vi "Signal.vi"() -> ()   [LabVIEW 2017]
uses:
  <vilib>/measure/NI_MABase.lvlib
panel:
  out "Waveform Chart":dynamicdata(graph)
  in  "sampling info":cluster{"Fs":dbl, "#s":dbl}={"Fs"=1000.0, "#s"=1000.0} {"Fs" format="%.2p"}
  out "data 2":waveform(dbl)(graph) caption="data"
  in  "Desviación\nEstandar":dbl=1.0 format="%.2p"
  in  "input cluster":T1={"amplitude"=2.0, "frequency"=10.0, "offset"=2.0, "square wave duty cycle (%)"=50.0, "reset signal"=FALSE, "signal type"=enum."Sine Wave", "phase"=0.0} {"phase" format="%.2p"; "square wave duty cycle (%)" format="%0.2f"; "offset" format="%0.2p"; "frequency" format="%0.2p"; "amplitude" format="%0.2p"}
  in  "device name":tag="myDAQ1"
  out "data":dynamicdata(graph)
  in  "stop":bool
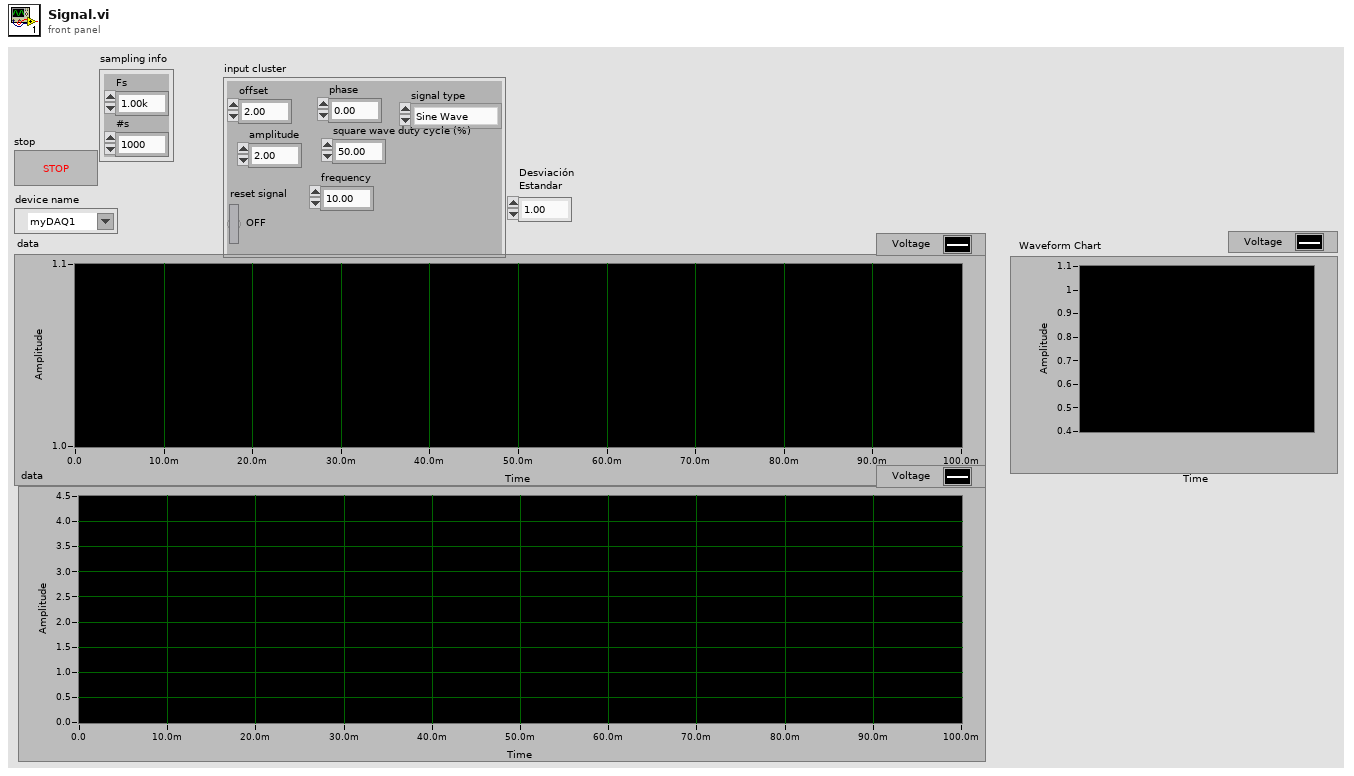
[diagram p1: front panel]
types:
  T1 = cluster{"amplitude":dbl, "frequency":dbl, "offset":dbl, "square wave duty cycle (%)":dbl, "reset signal":bool, "signal type":enum16{"Sine Wave", "Triangle Wave", "Square Wave", "Sawtooth Wave"}, "phase":dbl}
  T2 = enum16{"Sine Wave", "Triangle Wave", "Square Wave", "Sawtooth Wave"}
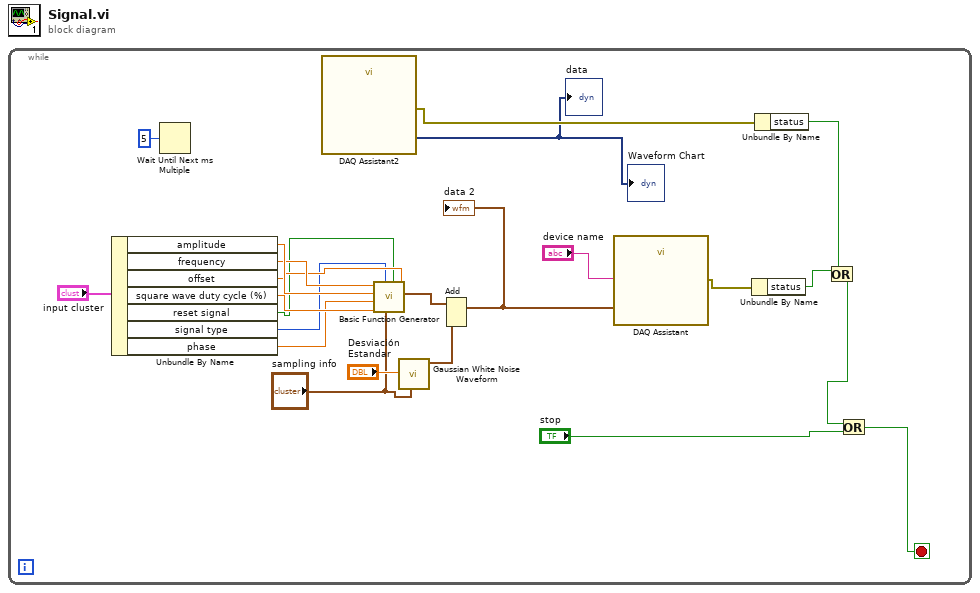
[diagram p0: block diagram]
diagram:
  n1 = while {
    stop <- w4 stop-if-true
    n2 = Unbundle By Name("input cluster") -> ("amplitude"=w21:dbl, "frequency"=w20:dbl, "offset"=w19:dbl, "square wave duty cycle (%)"=w18:dbl, "reset signal"=w17:bool, "signal type"=w16:T2, "phase"=w15:dbl)
    n3 = Wait Until Next ms Multiple(millisecond multiple=u32 5) -> ()  [unwired: 1 out]
    n4 = call "DAQ Assistant2"() -> ("data"=→"data" →"Waveform Chart":dynamicdata, "error out"=w5:errorcluster)  [unwired: 17 in, 1 out]
    n5 = call <vilib>:"Basic Function Generator.vi"("offset"=w19, "square wave duty cycle (%)"=w18, "reset signal"=w17, "sampling info"="sampling info", "signal type"=w16, "phase"=w15, "amplitude"=w21, "frequency"=w20) -> ("signal out"=w13:waveform(dbl))  [unwired: 1 in, 2 out]
    n6 = call <vilib>:"Gaussian White Noise Waveform.vi"("sampling info"="sampling info", "standard deviation"="Desviación\nEstandar") -> ("signal out"=w12:waveform(dbl))  [unwired: 8 in, 1 out]
    n7 = Add(1:w12, 2:w13) -> (0:w10:waveform(dbl))  [unwired: 1 in, 1 out]
    "data 2" <- w10
    n8 = call "DAQ Assistant"("data"=w10, "device name"="device name") -> ("error out"=w6:errorcluster)  [unwired: 16 in, 1 out]
    n9 = Unbundle By Name(w6) -> ("status"=w8:bool)
    n10 = Unbundle By Name(w5) -> ("status"=w7:bool)
    n11 = Or(x=w8, y=w7) -> (x .or. y?=w9:bool)
    n12 = Or(x=w9, y="stop") -> (x .or. y?=w4:bool)
  }
